vi "未命名 2.vi"(8 "错误输入（无错误）":errorcluster, 10 "Task Info.Accele Task":T1[](array[typedef]), 11 "TDMS in":refnum<k34>) -> (0 "错误输入（无错误）":errorcluster, 3 "TDMS out":refnum<k34>)   [LabVIEW 2011]
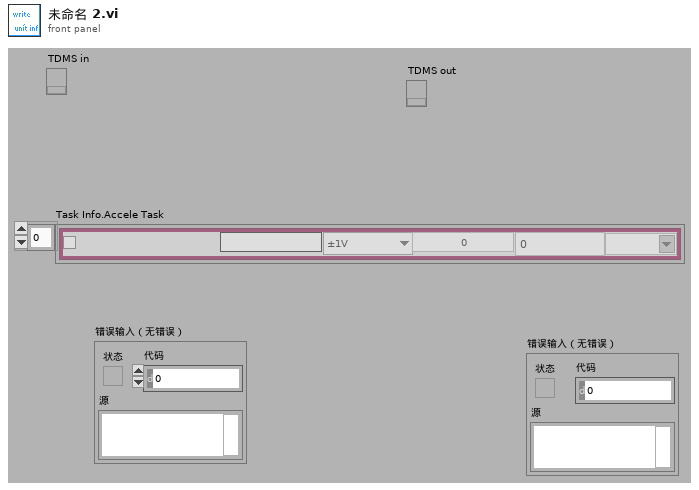
[diagram p1: front panel]
types:
  T1 = typedef "Acceleration Channel Config_Ctrls-某型振动实验台测试系统.ctl" = cluster{"Enable":bool, "Name":string, "range":enum16{"±1V", "±5V"}, "SensValue":dbl, "PhysicalName":string, "off":dbl, "Sensunits":string}
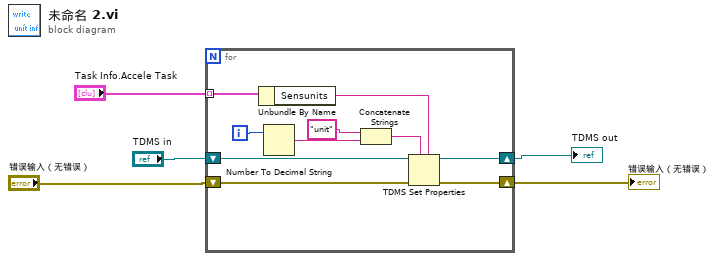
[diagram p0: block diagram]
diagram:
  n1 = for {
    tunnel: "Task Info.Accele Task" -> [w15] mode=indexing
    shift-right: [w12] -> w3
    shift-left: "TDMS in" -> [w13]
    shift-right: [w10] -> w1
    shift-left: "错误输入（无错误）" -> [w11]
    i -> [w9]
    n2 = Unbundle By Name(w15) -> ("Sensunits"=w14:string)
    n3 = Number To Decimal String(number=w9) -> (decimal integer string=w7:string)  [unwired: 1 out]
    n4 = Concatenate Strings("unit" ("字符串"), w7) -> (w8:string)
    n5 = TDMS Set Properties(5:w14, 7:w8, 8:w11, 11:w13) -> (0:w10:errorcluster, 3:w12:refnum<k34>)  [unwired: 4 out]
  }
  "TDMS out" <- w3
  "错误输入（无错误）" <- w1
